vi "Arm Button Case Handler.vi"(0 "Draw Bridge":bool=TRUE, 1 "Arm Drive Position":bool=TRUE, 2 "Portcullis":bool=TRUE, 3 "Sally Door":bool=TRUE, 4 "Harvest":bool=TRUE, 5 "Arm Up":bool=TRUE, 6 "Shoot Position":bool=TRUE, 7 "Arm Down":bool=TRUE, 9 "Roll Out":bool=TRUE, 11 "Current Arm State":T1=enum."Draw Bridge Arm Down") -> (14 "Arm state":T1=enum."Draw Bridge Arm Down")   [LabVIEW 2015]
uses:
  ArmStates.ctl
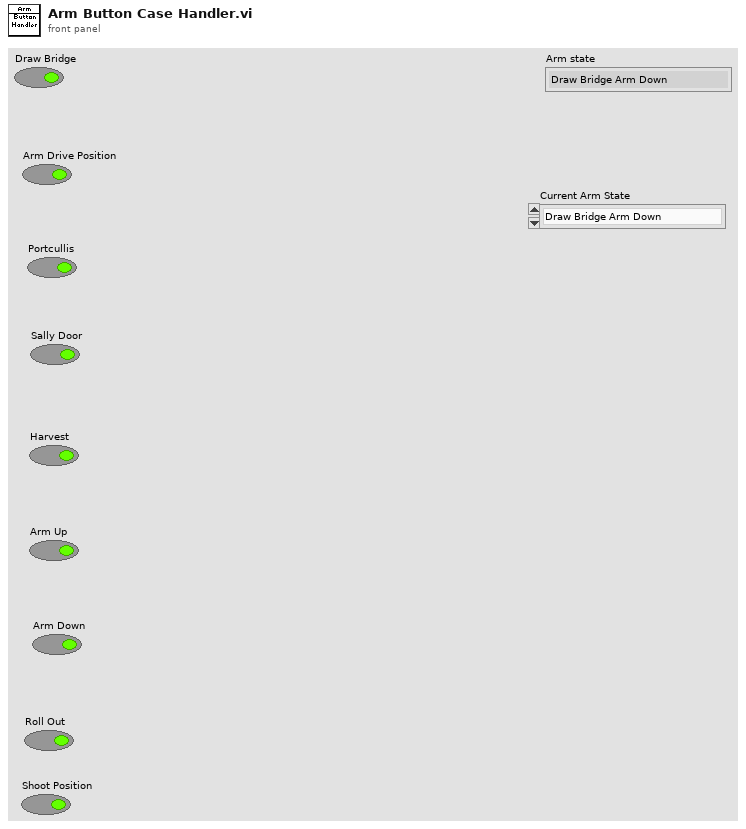
[diagram p1: front panel]
types:
  T1 = typedef "ArmStates.ctl" = enum16{"Arm Drive Position", "Shoot Position", "Roll Out", "Hic Up Rollers Off", "Draw Bridge Arm Down", "Harvest Back Down", "Harvest Hic up", "Portcullis", "Sally Door", "Harvest", "Arm Up", "Arm Down"}
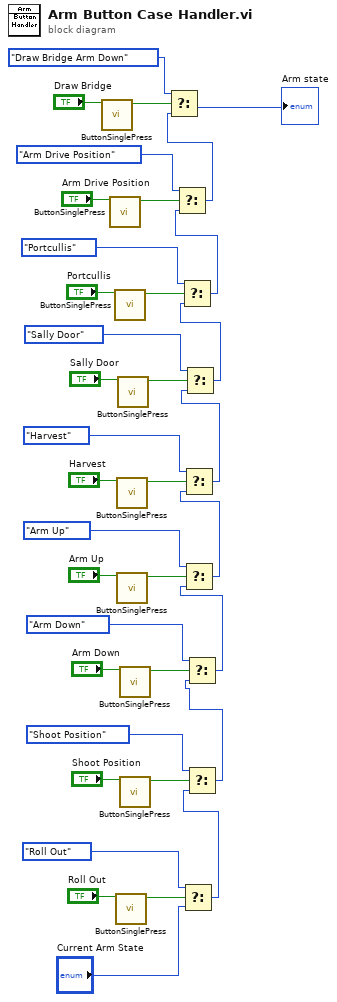
[diagram p0: block diagram]
diagram:
  n1 = call "ButtonSinglePress.vi"("Button In"="Draw Bridge") -> ("Button out"=w34:bool)  [unwired: 10 in]
  n2 = call "ButtonSinglePress.vi"("Button In"="Arm Drive Position") -> ("Button out"=w33:bool)  [unwired: 10 in]
  n3 = call "ButtonSinglePress.vi"("Button In"="Portcullis") -> ("Button out"=w28:bool)  [unwired: 10 in]
  n4 = call "ButtonSinglePress.vi"("Button In"="Roll Out") -> ("Button out"=w8:bool)  [unwired: 10 in]
  n5 = call "ButtonSinglePress.vi"("Button In"="Harvest") -> ("Button out"=w19:bool)  [unwired: 10 in]
  n6 = call "ButtonSinglePress.vi"("Button In"="Arm Up") -> ("Button out"=w18:bool)  [unwired: 10 in]
  n7 = call "ButtonSinglePress.vi"("Button In"="Sally Door") -> ("Button out"=w27:bool)  [unwired: 10 in]
  n8 = call "ButtonSinglePress.vi"("Button In"="Arm Down") -> ("Button out"=w11:bool)  [unwired: 10 in]
  n9 = call "ButtonSinglePress.vi"("Button In"="Shoot Position") -> ("Button out"=w5:bool)  [unwired: 10 in]
  n10 = Select(t=ArmStates."Roll Out" ("Arm State"), s=w8, f="Current Arm State") -> (s? t:f=w1:T1)
  n11 = Select(t=ArmStates."Shoot Position" ("Arm State"), s=w5, f=w1) -> (s? t:f=w2:T1)
  n12 = Select(t=ArmStates."Arm Down" ("Arm State"), s=w11, f=w2) -> (s? t:f=w10:T1)
  n13 = Select(t=ArmStates."Arm Up" ("Arm State"), s=w18, f=w10) -> (s? t:f=w15:T1)
  n14 = Select(t=ArmStates."Harvest" ("Arm State"), s=w19, f=w15) -> (s? t:f=w14:T1)
  n15 = Select(t=ArmStates."Sally Door" ("Arm State"), s=w27, f=w14) -> (s? t:f=w22:T1)
  n16 = Select(t=ArmStates."Portcullis" ("Arm State"), s=w28, f=w22) -> (s? t:f=w23:T1)
  n17 = Select(t=ArmStates."Arm Drive Position" ("Arm State"), s=w33, f=w23) -> (s? t:f=w24:T1)
  n18 = Select(t=ArmStates."Draw Bridge Arm Down" ("Arm State"), s=w34, f=w24) -> (s? t:f=→"Arm state":T1)
